vi "Add Status.vi"(10 "i":i32, 11 "New Status":string) -> (3 "Status history":string)   [LabVIEW 2020, in "Application.lvlib"]
uses:
  Application.lvlib
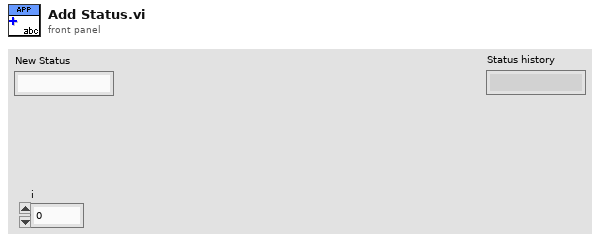
[diagram p1: front panel]
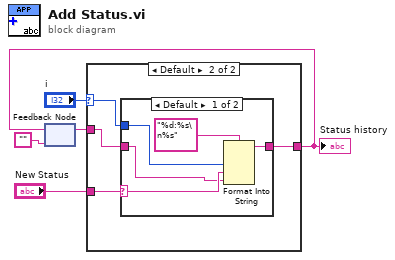
[diagram p0: block diagram]
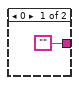
[diagram p2: hidden frame]
diagram:
  n1 = feedback #1("") -> (w2:string)
  n2 = case shown="Default" "i" {
    selector: "i" -> [_ w7]
    tunnel: "New Status" -> [_ w10]
    tunnel: ["" w9] -> w1
    tunnel: w2 -> [_ w8]
    frame 0 {
    }
    frame Default {
      n3 = case shown="Default" w10 {
        selector: w10 -> [w12 _]
        tunnel: [w14 w16] -> w9
        tunnel: w8 -> [w11 w16]
        tunnel: w7 -> [w13 _]
        frame Default {
          n4 = Format Into String(format string="%d:%s\n%s", w13, w12, w11) -> (resulting string=w14:string)  [unwired: 2 in, 1 out]
        }
        frame "" {
        }
      }
    }
  }
  "Status history" <- w1
  n5 = feedback-in #1(w1) -> ()
